vi "Save VI as Image.vi"() -> ()   [LabVIEW 2016]
panel:
  in  "VI path":path
  in  "Image path":path
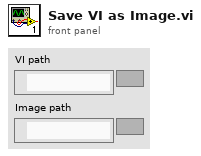
[diagram p1: front panel]
types:
  T1 = typedef "imagedata.ctl" = cluster{"image type":i32, "image depth":i32, "image":u8[], "mask":u8[], "colors":u32[], "Rectangle":cluster{"left":i16, "top":i16, "right":i16, "bottom":i16}}
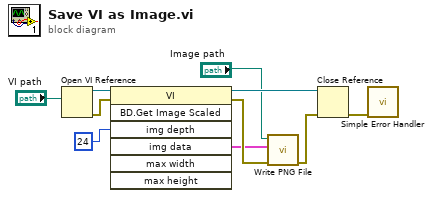
[diagram p0: block diagram]
diagram:
  n1 = Open VI Reference(vi path="VI path") -> (vi reference=w9:refnum<vi>, error out=w5:errorcluster)  [unwired: 5 in]
  n2 = invoke class="VI" method="BD.Get Image Scaled"(reference=w9, error in=w5, "img depth"=24 ("Image Depth")) -> (reference out=w6:refnum<vi>, error out=w10:errorcluster, "img data"=w7:T1)  [unwired: 4 in, 4 out]
  n3 = call <vilib>:"Write PNG File.vi"("error in (no error)"=w10, "image data"=w7, "path to PNG file"="Image path") -> ("error out"=w4:errorcluster)  [unwired: 7 in, 1 out]
  n4 = Close Reference(reference=w6, error in (no error)=w4) -> (error out=w3:errorcluster)
  n5 = call <vilib>:"Simple Error Handler.vi"("error in (no error)"=w3) -> ()  [unwired: 4 in, 5 out]
